vi "Peak Params.vi"(6 "ID (Profile)":string="Profile", 7 "PEAK params":T1, 8 "error in (no error)":errorcluster, 11 "Profile NO":u8=1 min=1 max=50 step=1) -> (0 "error out":errorcluster, 2 "wchitch params":string, 3 "params array out":string[](array[string]))   [LabVIEW 2019, in "STAV lib.lvlib"]
uses:
  STAV lib.lvlib
  Peak params.ctl
  Param Units.ctl
  Param Direction.ctl
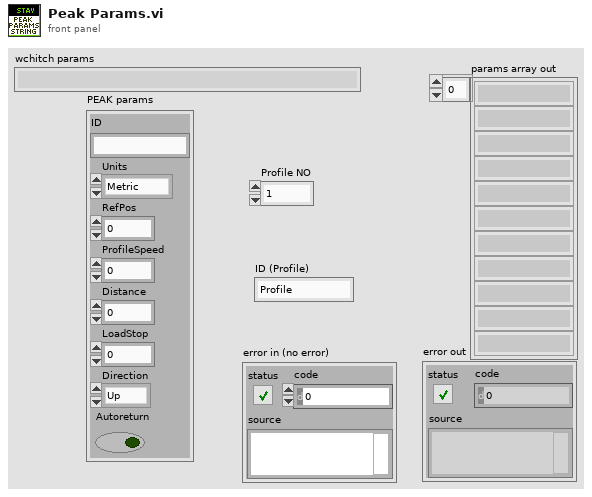
[diagram p1: front panel]
types:
  T1 = typedef "STAV lib.lvlib/Peak params.ctl" = cluster{"ID":string, "Units":T2, "RefPos":dbl, "ProfileSpeed":dbl, "Distance":dbl, "LoadStop":dbl, "Direction":T3, "Autoreturn":bool}
  T2 = typedef "STAV lib.lvlib/Param Units.ctl" = enum16{"Metric", "Imperial"}
  T3 = typedef "STAV lib.lvlib/Param Direction.ctl" = enum16{"Up", "Down", "Left", "Right"}
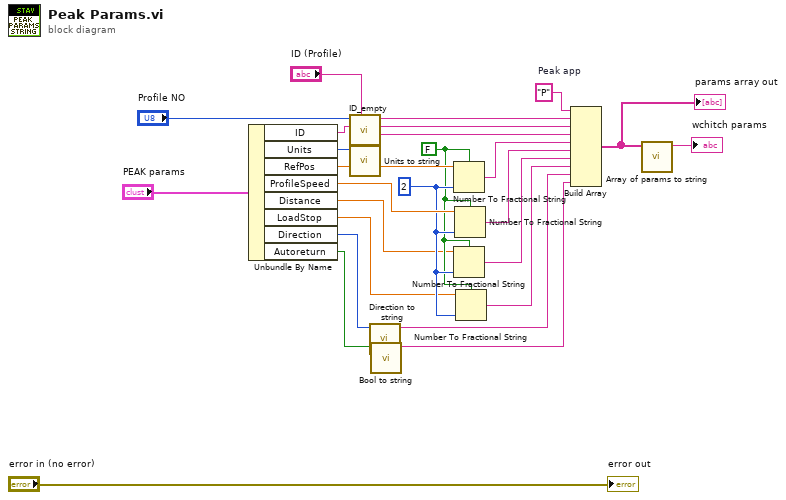
[diagram p0: block diagram]
diagram:
  w17 = i16 2 ("precision (6)")
  w16 = FALSE ("use system decimal point (T)")
  w25 = "P"  # Peak app
  n1 = Unbundle By Name("PEAK params") -> ("ID"=w5:string, "Units"=w22:T2, "RefPos"=w21:dbl, "ProfileSpeed"=w18:dbl, "Distance"=w15:dbl, "LoadStop"=w14:dbl, "Direction"=w13:T3, "Autoreturn"=w12:bool)
  n2 = call "ID_empty.vi"("ID (Profile)"="ID (Profile)", "ID in"=w5, "Profile NO"="Profile NO") -> ("ID out"=w4:string, "Profile NO out"=w6:string)  [unwired: 7 in]
  n3 = call "Units to string.vi"("Units"=w22) -> ("Peak app"=w20:string)  [unwired: 10 in]
  n4 = call "Direction to string.vi"("Direction"=w13) -> ("Peak app"=w8:string)  [unwired: 10 in]
  n5 = call "Bool to string.vi"("Autoreturn"=w12) -> ("Peak app"=w7:string)  [unwired: 10 in]
  n6 = Number To Fractional String(use system decimal point (T)=w16, number=w21, precision (6)=w17) -> (F-format string=w19:string)  [unwired: 1 in]
  n7 = Number To Fractional String(use system decimal point (T)=w16, number=w15, precision (6)=w17) -> (F-format string=w10:string)  [unwired: 1 in]
  n8 = Number To Fractional String(use system decimal point (T)=w16, number=w18, precision (6)=w17) -> (F-format string=w11:string)  [unwired: 1 in]
  n9 = Number To Fractional String(use system decimal point (T)=w16, number=w14, precision (6)=w17) -> (F-format string=w9:string)  [unwired: 1 in]
  n10 = Build Array(w25, w6, w4, w20, w19, w11, w10, w9, w8, w7) -> (w3:string[])
  "params array out" <- w3
  n11 = call "Array of params to string.vi"("Array"=w3) -> ("String"=→"wchitch params":string)  [unwired: 10 in]
  "error out" <- "error in (no error)"
